vi "Lab Panel V5.26.vi"() -> ()   [LabVIEW 2017] (continued)
                        n2902 = local write "MAIL SETTINGS"(w5260) -> ()
                      }
                    }
                  }
                }
              }
              frame #1 {
                # "mail report"
                n2903 = stacked-sequence {
                  seq-local: [_ w5320 _ _] -> [_ _ _ w5510]
                  seq-local: [_ _ w5423 _] -> [_ _ _ w5500]
                  seq-local: [w5287 _ _ _] -> [_ w5337 _ _]
                  seq-local: [w5286 _ _ _] -> [_ w5336 _ _]
                  seq-local: [w5284 _ _ _] -> [_ w5334 _ _]
                  seq-local: [w5285 _ _ _] -> [_ w5335 _ _]
                  seq-local: [w5283 _ _ _] -> [_ w5333 _ _]
                  seq-local: [w5282 _ _ _] -> [_ w5328 _ _]
                  seq-local: [w5281 _ _ _] -> [_ w5329 _ _]
                  seq-local: [w5280 _ _ _] -> [_ w5330 _ _]
                  seq-local: [w5279 _ _ _] -> [_ w5331 _ _]
                  seq-local: [w5278 _ _ _] -> [_ w5332 _ _]
                  tunnel: w5277 -> [_ _ _ w5511]
                  tunnel: w5276 -> [_ _ _ w5494]
                  tunnel: w5275 -> [_ _ _ w5508]
                  tunnel: w5274 -> [_ _ _ w5507]
                  tunnel: w5273 -> [w5318 _ _ w5502]
                  tunnel: w5272 -> [_ _ w5453 _]
                  tunnel: w5271 -> [_ _ w5450 _]
                  tunnel: w5270 -> [_ _ w5449 _]
                  tunnel: w5269 -> [_ _ w5448 _]
                  tunnel: w5268 -> [_ _ w5447 _]
                  tunnel: w5267 -> [_ _ w5446 _]
                  tunnel: w5266 -> [_ _ w5445 _]
                  tunnel: w5265 -> [_ _ w5444 _]
                  tunnel: w5264 -> [_ _ w5443 _]
                  tunnel: w5263 -> [_ _ w5442 _]
                  frame #0 {
                    n2904 = case shown="False" w5318 {
                      frame False {
                        n2905 = local write "mail control"("") -> ()
                      }
                      frame True {
                      }
                    }
                    n2906 = local read "SET LAB01-1"() -> (w5317:T5)
                    n2907 = local read "SET LAB01-2"() -> (w5316:T5)
                    n2908 = local read "SET LAB02-1"() -> (w5315:T5)
                    n2909 = local read "SET LAB02-2"() -> (w5314:T5)
                    n2910 = local read "SET LAB03-1"() -> (w5313:T5)
                    n2911 = local read "SET LAB04-1"() -> (w5311:T5)
                    n2912 = local read "SET LAB05-1"() -> (w5309:T5)
                    n2913 = local read "SET LAB03-2"() -> (w5312:T5)
                    n2914 = local read "SET LAB04-2"() -> (w5310:T5)
                    n2915 = local read "SET LAB05-2"() -> (w5308:T5)
                    n2916 = Unbundle(w5313) -> ("DESCRIPTION"=w5293:string)  [unwired: 4 out]
                    n2917 = Unbundle(w5312) -> ("DESCRIPTION"=w5292:string)  [unwired: 4 out]
                    n2918 = Unbundle(w5311) -> ("DESCRIPTION"=w5291:string)  [unwired: 4 out]
                    n2919 = Unbundle(w5308) -> ("DESCRIPTION"=w5288:string)  [unwired: 4 out]
                    n2920 = Unbundle(w5314) -> ("DESCRIPTION"=w5294:string)  [unwired: 4 out]
                    n2921 = Unbundle(w5310) -> ("DESCRIPTION"=w5290:string)  [unwired: 4 out]
                    n2922 = Unbundle(w5317) -> ("DESCRIPTION"=w5306:string)  [unwired: 4 out]
                    n2923 = Unbundle(w5315) -> ("DESCRIPTION"=w5295:string)  [unwired: 4 out]
                    n2924 = Unbundle(w5309) -> ("DESCRIPTION"=w5289:string)  [unwired: 4 out]
                    n2925 = Unbundle(w5316) -> ("DESCRIPTION"=w5296:string)  [unwired: 4 out]
                    n2926 = Concatenate Strings("[LAB05-2/", w5288) -> (w5278:string)
                    n2927 = Concatenate Strings("[LAB05-1/", w5289) -> (w5279:string)
                    n2928 = Concatenate Strings("[LAB04-2/", w5290) -> (w5280:string)
                    n2929 = Concatenate Strings("[LAB03-2/", w5292) -> (w5282:string)
                    n2930 = Concatenate Strings("[LAB04-1/", w5291) -> (w5281:string)
                    n2931 = Concatenate Strings("[LAB03-1/", w5293) -> (w5283:string)
                    n2932 = Concatenate Strings("[LAB01-2/", w5296) -> (w5286:string)
                    n2933 = Concatenate Strings("[LAB02-2/", w5294) -> (w5284:string)
                    n2934 = Concatenate Strings("[LAB01-1/", w5306) -> (w5287:string)
                    n2935 = Concatenate Strings("[LAB02-1/", w5295) -> (w5285:string)
                  }
                  frame #1 {
                    w5341 = "/"
                    w5342 = 2.0
                    n2936 = local read "DISP LAB01-2"() -> (w5421:T4)
                    n2937 = local read "DISP LAB01-1"() -> (w5422:T4)
                    n2938 = local read "DISP LAB02-1"() -> (w5420:T4)
                    n2939 = local read "DISP LAB03-2"() -> (w5417:T4)
                    n2940 = local read "DISP LAB02-2"() -> (w5419:T4)
                    n2941 = local read "DISP LAB03-1"() -> (w5418:T4)
                    n2942 = local read "DISP LAB04-2"() -> (w5415:T4)
                    n2943 = local read "DISP LAB04-1"() -> (w5416:T4)
                    n2944 = local read "DISP LAB05-1"() -> (w5414:T4)
                    n2945 = local read "DISP LAB05-2"() -> (w5413:T4)
                    n2946 = Unbundle(w5421) -> ("CYCLE"=w5405:dbl, "MINS"=w5404:dbl, "STATUS"=w5401:string)
                    n2947 = Unbundle(w5422) -> ("CYCLE"=w5410:dbl, "MINS"=w5409:dbl, "STATUS"=w5406:string)
                    n2948 = Unbundle(w5420) -> ("CYCLE"=w5398:dbl, "MINS"=w5397:dbl, "STATUS"=w5396:string)
                    n2949 = Unbundle(w5417) -> ("CYCLE"=w5385:dbl, "MINS"=w5384:dbl, "STATUS"=w5381:string)
                    n2950 = Unbundle(w5418) -> ("CYCLE"=w5390:dbl, "MINS"=w5389:dbl, "STATUS"=w5386:string)
                    n2951 = Unbundle(w5419) -> ("CYCLE"=w5395:dbl, "MINS"=w5394:dbl, "STATUS"=w5391:string)
                    n2952 = Unbundle(w5416) -> ("CYCLE"=w5380:dbl, "MINS"=w5379:dbl, "STATUS"=w5376:string)
                    n2953 = Unbundle(w5415) -> ("CYCLE"=w5375:dbl, "MINS"=w5374:dbl, "STATUS"=w5371:string)
                    n2954 = Unbundle(w5414) -> ("CYCLE"=w5370:dbl, "MINS"=w5369:dbl, "STATUS"=w5366:string)
                    n2955 = Unbundle(w5413) -> ("CYCLE"=w5412:dbl, "MINS"=w5411:dbl, "STATUS"=w5363:string)
                    n2956 = Number To Decimal String(number=w5398) -> (decimal integer string=w5400:string)  [unwired: 1 in]
                    n2957 = Number To Decimal String(number=w5395) -> (decimal integer string=w5393:string)  [unwired: 1 in]
                    n2958 = Number To Decimal String(number=w5390) -> (decimal integer string=w5388:string)  [unwired: 1 in]
                    n2959 = Number To Decimal String(number=w5405) -> (decimal integer string=w5403:string)  [unwired: 1 in]
                    n2960 = Number To Decimal String(number=w5385) -> (decimal integer string=w5383:string)  [unwired: 1 in]
                    n2961 = Number To Decimal String(number=w5410) -> (decimal integer string=w5408:string)  [unwired: 1 in]
                    n2962 = Number To Decimal String(number=w5412) -> (decimal integer string=w5365:string)  [unwired: 1 in]
                    n2963 = Number To Decimal String(number=w5380) -> (decimal integer string=w5378:string)  [unwired: 1 in]
                    n2964 = Number To Decimal String(number=w5375) -> (decimal integer string=w5373:string)  [unwired: 1 in]
                    n2965 = Number To Decimal String(number=w5370) -> (decimal integer string=w5368:string)  [unwired: 1 in]
                    n2966 = Number To Fractional String(number=w5397, precision (6)=w5342) -> (F-format string=w5399:string)  [unwired: 2 in]
                    n2967 = Number To Fractional String(number=w5384, precision (6)=w5342) -> (F-format string=w5382:string)  [unwired: 2 in]
                    n2968 = Number To Fractional String(number=w5394, precision (6)=w5342) -> (F-format string=w5392:string)  [unwired: 2 in]
                    n2969 = Number To Fractional String(number=w5389, precision (6)=w5342) -> (F-format string=w5387:string)  [unwired: 2 in]
                    n2970 = Number To Fractional String(number=w5374, precision (6)=w5342) -> (F-format string=w5372:string)  [unwired: 2 in]
                    n2971 = Number To Fractional String(number=w5379, precision (6)=w5342) -> (F-format string=w5377:string)  [unwired: 2 in]
                    n2972 = Number To Fractional String(number=w5404, precision (6)=w5342) -> (F-format string=w5402:string)  [unwired: 2 in]
                    n2973 = Number To Fractional String(number=w5369, precision (6)=w5342) -> (F-format string=w5367:string)  [unwired: 2 in]
                    n2974 = Number To Fractional String(number=w5409, precision (6)=w5342) -> (F-format string=w5407:string)  [unwired: 2 in]
                    n2975 = Number To Fractional String(number=w5411, precision (6)=w5342) -> (F-format string=w5364:string)  [unwired: 2 in]
                    n2976 = Concatenate Strings(w5341, w5383, w5341, w5382, w5341, w5381) -> (w5357:string)
                    n2977 = Concatenate Strings(w5341, w5378, w5341, w5377, w5341, w5376) -> (w5356:string)
                    n2978 = Concatenate Strings(w5341, w5373, w5341, w5372, w5341, w5371) -> (w5355:string)
                    n2979 = Concatenate Strings(w5341, w5368, w5341, w5367, w5341, w5366) -> (w5354:string)
                    n2980 = Concatenate Strings(w5341, w5365, w5341, w5364, w5341, w5363) -> (w5353:string)
                    n2981 = Concatenate Strings(w5341, w5408, w5341, w5407, w5341, w5406) -> (w5362:string)
                    n2982 = Concatenate Strings(w5341, w5388, w5341, w5387, w5341, w5386) -> (w5358:string)
                    n2983 = Concatenate Strings(w5341, w5403, w5341, w5402, w5341, w5401) -> (w5361:string)
                    n2984 = Concatenate Strings(w5341, w5400, w5341, w5399, w5341, w5396) -> (w5360:string)
                    n2985 = Concatenate Strings(w5341, w5393, w5341, w5392, w5341, w5391) -> (w5359:string)
                    n2986 = Concatenate Strings("]", "\r") -> (w5338:string)
                    n2987 = Concatenate Strings(w5333, w5358, w5338) -> (w5348:string)
                    n2988 = Concatenate Strings(w5335, w5360, w5338) -> (w5350:string)
                    n2989 = Concatenate Strings(w5334, w5359, w5338) -> (w5349:string)
                    n2990 = Concatenate Strings(w5330, w5355, w5338) -> (w5345:string)
                    n2991 = Concatenate Strings(w5331, w5354, w5338) -> (w5346:string)
                    n2992 = Concatenate Strings(w5329, w5356, w5338) -> (w5344:string)
                    n2993 = Concatenate Strings(w5328, w5357, w5338) -> (w5343:string)
                    n2994 = Concatenate Strings(w5332, w5353, w5338) -> (w5347:string)
                    n2995 = Concatenate Strings(w5336, w5361, w5338) -> (w5351:string)
                    n2996 = Concatenate Strings(w5337, w5362, w5338) -> (w5352:string)
                    n2997 = Concatenate Strings(w5352, w5351, w5350, w5349, w5348, w5343, w5344, w5345, w5346, w5347) -> (w5321:string)
                    n2998 = Concatenate Strings("[PANEL/", "DESC/", "CYCLES/", "MINS/", "STATUS]", "\r", w5321) -> (w5320:string)
                    "MAIL REPORT" <- w5320
                    n2999 = global write "Global display 3.vi" "log all"(w5320) -> ()
                  }
                  frame #2 {
                    w5451 = "END"
                    n3000 = local read "mail control"() -> (w5452:string)
                    n3001 = case shown="False" w5447 {
                      tunnel: w5452 -> [w5476 _]
                      tunnel: w5451 -> [w5475 _]
                      tunnel: [w5474 FALSE] -> w5437
                      frame False {
                        n3002 = Equal?(x=w5476, y=w5475) -> (x = y?=w5474:bool)
                      }
                      frame True {
                      }
                    }
                    n3003 = case shown="False" w5453 {
                      tunnel: w5452 -> [w5492 _]
                      tunnel: w5451 -> [w5491 _]
                      tunnel: [w5490 FALSE] -> w5441
                      frame False {
                        n3004 = Equal?(x=w5492, y=w5491) -> (x = y?=w5490:bool)
                      }
                      frame True {
                      }
                    }
                    n3005 = case shown="False" w5450 {
                      tunnel: w5452 -> [w5488 _]
                      tunnel: w5451 -> [w5487 _]
                      tunnel: [w5486 FALSE] -> w5440
                      frame False {
                        n3006 = Equal?(x=w5488, y=w5487) -> (x = y?=w5486:bool)
                      }
                      frame True {
                      }
                    }
                    n3007 = case shown="False" w5448 {
                      tunnel: w5452 -> [w5480 _]
                      tunnel: w5451 -> [w5479 _]
                      tunnel: [w5478 FALSE] -> w5438
                      frame False {
                        n3008 = Equal?(x=w5480, y=w5479) -> (x = y?=w5478:bool)
                      }
                      frame True {
                      }
                    }
                    n3009 = case shown="False" w5449 {
                      tunnel: w5452 -> [w5484 _]
                      tunnel: w5451 -> [w5483 _]
                      tunnel: [w5482 FALSE] -> w5439
                      frame False {
                        n3010 = Equal?(x=w5484, y=w5483) -> (x = y?=w5482:bool)
                      }
                      frame True {
                      }
                    }
                    n3011 = Or(x=w5439, y=w5438) -> (x .or. y?=w5430:bool)
                    n3012 = Or(x=w5441, y=w5440) -> (x .or. y?=w5431:bool)
                    n3013 = Or(x=w5431, y=w5430) -> (x .or. y?=w5426:bool)
                    n3014 = case shown="False" w5443 {
                      tunnel: w5452 -> [w5460 _]
                      tunnel: w5451 -> [w5459 _]
                      tunnel: [w5458 FALSE] -> w5432
                      frame False {
                        n3015 = Equal?(x=w5460, y=w5459) -> (x = y?=w5458:bool)
                      }
                      frame True {
                      }
                    }
                    n3016 = case shown="False" w5442 {
                      tunnel: w5452 -> [w5456 _]
                      tunnel: w5451 -> [w5455 _]
                      tunnel: [w5454 FALSE] -> w5436
                      frame False {
                        n3017 = Equal?(x=w5456, y=w5455) -> (x = y?=w5454:bool)
                      }
                      frame True {
                      }
                    }
                    n3018 = case shown="False" w5444 {
                      tunnel: w5452 -> [w5464 _]
                      tunnel: w5451 -> [w5463 _]
                      tunnel: [w5462 FALSE] -> w5433
                      frame False {
                        n3019 = Equal?(x=w5464, y=w5463) -> (x = y?=w5462:bool)
                      }
                      frame True {
                      }
                    }
                    n3020 = case shown="False" w5446 {
                      tunnel: w5452 -> [w5472 _]
                      tunnel: w5451 -> [w5471 _]
                      tunnel: [w5470 FALSE] -> w5435
                      frame False {
                        n3021 = Equal?(x=w5472, y=w5471) -> (x = y?=w5470:bool)
                      }
                      frame True {
                      }
                    }
                    n3022 = case shown="False" w5445 {
                      tunnel: w5452 -> [w5468 _]
                      tunnel: w5451 -> [w5467 _]
                      tunnel: [w5466 FALSE] -> w5434
                      frame False {
                        n3023 = Equal?(x=w5468, y=w5467) -> (x = y?=w5466:bool)
                      }
                      frame True {
                      }
                    }
                    n3024 = Or(x=w5435, y=w5434) -> (x .or. y?=w5429:bool)
                    n3025 = Or(x=w5433, y=w5432) -> (x .or. y?=w5428:bool)
                    n3026 = Or(x=w5436, y=w5437) -> (x .or. y?=w5424:bool)
                    n3027 = Or(x=w5429, y=w5428) -> (x .or. y?=w5427:bool)
                    n3028 = Or(x=w5426, y=w5427) -> (x .or. y?=w5425:bool)
                    n3029 = Or(x=w5425, y=w5424) -> (x .or. y?=w5423:bool)
                  }
                  frame #3 {
                    n3030 = local read "on loops"() -> (w5506:dbl)
                    n3031 = local read "jig cycle"() -> (w5503:dbl)
                    n3032 = local read "Send Mail Now"() -> (w5497:bool)
                    n3033 = Add(x=w5506, y=5.0) -> (x+y=w5504:dbl)
                    n3034 = Equal?(x=w5503, y=w5504) -> (x = y?=w5498:bool)
                    n3035 = And(x=w5498, y=w5497) -> (x .and. y?=w5496:bool)
                    n3036 = And(x=w5502, y=w5498) -> (x .and. y?=w5501:bool)
                    n3037 = And(x=w5501, y=w5500) -> (x .and. y?=w5499:bool)
                    n3038 = Or(x=w5499, y=w5496) -> (x .or. y?=w5495:bool)
                    n3039 = case shown="True" w5495 {
                      tunnel: w5511 -> [_ w5517]
                      tunnel: w5510 -> [_ w5516]
                      tunnel: "Lab Panel Test Status" -> [_ w5515]
                      tunnel: w5508 -> [_ w5514]
                      tunnel: w5507 -> [_ w5513]
                      tunnel: w5494 -> [_ w5512]
                      frame False {
                      }
                      frame True {
                        n3040 = stacked-sequence {
                          tunnel: w5517 -> [w5525 _]
                          tunnel: w5516 -> [w5524 _]
                          tunnel: w5515 -> [w5523 _]
                          tunnel: w5514 -> [w5522 _]
                          tunnel: w5513 -> [w5521 _]
                          tunnel: w5512 -> [w5520 _]
                          frame #0 {
                            n3041 = call "Lab Send Mail Test.vi"("TO:"=w5525, "subject"=w5523, "from"=w5521, "out going server"=w5522, "message"=w5524) -> ("error out"=w5519:errorcluster)  [unwired: 10 in]
                            n3042 = Bundle(cluster=w5520, "mail error"=w5519) -> (w5518:T7)  [unwired: 6 in]
                            n3043 = local write "MAIL SETTINGS"(w5518) -> ()
                          }
                          frame #1 {
                            n3044 = local write "mail control"("") -> ()
                            n3045 = local write "Send Mail Now"(FALSE) -> ()
                          }
                        }
                      }
                    }
                  }
                }
              }
            }
          }
          frame #20 {
            # "save jig cycle values once all run switches are off"
            n3046 = stacked-sequence {
              tunnel: w5537 -> [_ w5566]
              tunnel: w5536 -> [_ w5565]
              tunnel: w5535 -> [_ w5564]
              tunnel: w5534 -> [_ w5563]
              tunnel: w5533 -> [_ w5562]
              tunnel: w5532 -> [_ w5561]
              tunnel: w5531 -> [_ w5560]
              tunnel: w5530 -> [_ w5559]
              tunnel: w5529 -> [_ w5558]
              tunnel: w5528 -> [_ w5557]
              frame #0 {
              }
              frame #1 {
                n3047 = Not(x=w5557) -> (.not. x?=w5540:bool)
                n3048 = Not(x=w5565) -> (.not. x?=w5555:bool)
                n3049 = Not(x=w5562) -> (.not. x?=w5550:bool)
                n3050 = Not(x=w5560) -> (.not. x?=w5546:bool)
                n3051 = Not(x=w5558) -> (.not. x?=w5542:bool)
                n3052 = Not(x=w5566) -> (.not. x?=w5556:bool)
                n3053 = Not(x=w5564) -> (.not. x?=w5554:bool)
                n3054 = Not(x=w5561) -> (.not. x?=w5548:bool)
                n3055 = Not(x=w5563) -> (.not. x?=w5552:bool)
                n3056 = Not(x=w5559) -> (.not. x?=w5544:bool)
                n3057 = local read "Save JC"() -> (w5568:bool)
                n3058 = And(x=w5556, y=w5555) -> (x .and. y?=w5553:bool)
                n3059 = And(x=w5553, y=w5554) -> (x .and. y?=w5551:bool)
                n3060 = And(x=w5551, y=w5552) -> (x .and. y?=w5549:bool)
                n3061 = And(x=w5549, y=w5550) -> (x .and. y?=w5547:bool)
                n3062 = And(x=w5547, y=w5548) -> (x .and. y?=w5545:bool)
                n3063 = And(x=w5545, y=w5546) -> (x .and. y?=w5543:bool)
                n3064 = And(x=w5543, y=w5544) -> (x .and. y?=w5541:bool)
                n3065 = And(x=w5541, y=w5542) -> (x .and. y?=w5539:bool)
                n3066 = And(x=w5539, y=w5540) -> (x .and. y?=w5538:bool)
                n3067 = And(x=w5538, y=w5568) -> (x .and. y?=w5567:bool)
                n3068 = case shown="True" w5567 {
                  tunnel: w5538 -> [w5569 _]
                  frame False {
                    n3069 = case shown="False" w5569 {
                      frame False {
                        n3070 = local write "Save JC"(TRUE) -> ()
                      }
                      frame True {
                      }
                    }
                  }
                  frame True {
                    n3071 = stacked-sequence {
                      frame #0 {
                        n3072 = String To Path(string="c:\\crabtree\\Jig Cycles\\") -> (path=w5581:path)
                        n3073 = Build Path(base path=w5581, name or relative path="jigcycles.bin") -> (appended path=w5579:path)
                        n3074 = Create Folder(path (use dialog)=w5581) -> (error out=w5583:errorcluster)  [unwired: 2 in, 2 out]
                        n3075 = local read "JIG RELAY CYCLES"() -> (w5573:T8)
                        n3076 = call <vilib>:"Clear Errors.vi"("error in (no error)"=w5583) -> ()  [unwired: 5 in, 2 out]
                        n3077 = local write "Save JC"(FALSE) -> ()
                        n3078 = Open/Create/Replace File(file path (use dialog)=w5579, operation (0:open)=T17."replace or create") -> (refnum out=w5577:refnum<file>, error out=w5578:errorcluster)  [unwired: 4 in, 1 out]
                        n3079 = Write to Binary File(file (use dialog)=w5577, data=w5573, error in=w5578) -> (refnum out=w5576:refnum<file>, error out=w5575:errorcluster)  [unwired: 3 in, 1 out]
                        n3080 = Close File(refnum=w5576, error in=w5575) -> (error out=w5574:errorcluster)  [unwired: 1 out]
                        n3081 = local write "data file error"(w5574) -> ()
                      }
                      frame #1 {
                        n3082 = local read "JIG RELAY CYCLES"() -> (w5606:T8)
                        n3083 = Unbundle By Name(w5606) -> ("LAB01-1"=w5601:dbl, "LAB01-2"=w5600:dbl, "LAB02-1"=w5598:dbl, "LAB02-2"=w5597:dbl, "LAB03-1"=w5595:dbl, "LAB03-2"=w5592:dbl, "LAB04-1"=w5591:dbl, "LAB04-2"=w5589:dbl, "LAB05-1"=w5587:dbl, "LAB05-2"=w5585:dbl)
                        n3084 = stacked-sequence {
                          tunnel: w5601 -> [w5609 _ _ _ _ _ _ _ _ _]
                          tunnel: 1000000 -> [w5612 w5622 w5632 w5642 w5652 w5662 w5672 w5682 w5692 w5702]
                          tunnel: [w5610 _ _ _ _ _ _ _ _ _] -> w5604
                          tunnel: "TEST STATION HAS REACHED 1 MILLION CYCLES, REPLACE  CONTROL RELAYS" -> [w5608 w5620 w5630 w5640 w5650 w5660 w5670 w5680 w5690 w5700]
                          tunnel: [_ w5619 _ _ _ _ _ _ _ _] -> w5602
                          tunnel: w5600 -> [_ w5618 _ _ _ _ _ _ _ _]
                          tunnel: [_ _ w5629 _ _ _ _ _ _ _] -> w5599
                          tunnel: w5598 -> [_ _ w5628 _ _ _ _ _ _ _]
                          tunnel: w5597 -> [_ _ _ w5639 _ _ _ _ _ _]
                          tunnel: [_ _ _ w5638 _ _ _ _ _ _] -> w5596
                          tunnel: w5595 -> [_ _ _ _ w5649 _ _ _ _ _]
                          tunnel: [_ _ _ _ w5648 _ _ _ _ _] -> w5594
                          tunnel: [_ _ _ _ _ w5659 _ _ _ _] -> w5593
                          tunnel: w5592 -> [_ _ _ _ _ w5658 _ _ _ _]
                          tunnel: w5591 -> [_ _ _ _ _ _ w5669 _ _ _]
                          tunnel: [_ _ _ _ _ _ w5668 _ _ _] -> w5590
                          tunnel: w5589 -> [_ _ _ _ _ _ _ w5679 _ _]
                          tunnel: [_ _ _ _ _ _ _ w5678 _ _] -> w5588
                          tunnel: w5587 -> [_ _ _ _ _ _ _ _ w5689 _]
                          tunnel: [_ _ _ _ _ _ _ _ w5688 _] -> w5586
                          tunnel: w5585 -> [_ _ _ _ _ _ _ _ _ w5699]
                          tunnel: [_ _ _ _ _ _ _ _ _ w5698] -> w5584
                          frame #0 {
                            n3085 = Greater?(x=w5609, y=w5612) -> (0:w5611:bool)
                            n3086 = case shown="True" w5611 {
                              tunnel: [w5613 0] -> w5610
                              tunnel: w5609 -> [w5613 _]
                              tunnel: w5608 -> [_ w5614]
                              frame False {
                              }
                              frame True {
                                n3087 = Concatenate Strings("LA01-1 ", w5614) -> (w5617:string)
                                n3088 = One Button Dialog(message=w5617) -> ()  [unwired: 1 in, 1 out]
                              }
                            }
                          }
                          frame #1 {
                            n3089 = Greater?(x=w5618, y=w5622) -> (0:w5621:bool)
                            n3090 = case shown="True" w5621 {
                              tunnel: [w5623 0] -> w5619
                              tunnel: w5618 -> [w5623 _]
                              tunnel: w5620 -> [_ w5624]
                              frame False {
                              }
                              frame True {
                                n3091 = Concatenate Strings("LA01-2 ", w5624) -> (w5627:string)
                                n3092 = One Button Dialog(message=w5627) -> ()  [unwired: 1 in, 1 out]
                              }
                            }
                          }
                          frame #2 {
                            n3093 = Greater?(x=w5628, y=w5632) -> (0:w5631:bool)
                            n3094 = case shown="True" w5631 {
                              tunnel: [w5633 0] -> w5629
                              tunnel: w5628 -> [w5633 _]
                              tunnel: w5630 -> [_ w5634]
                              frame False {
                              }
                              frame True {
                                n3095 = Concatenate Strings("LA02-1 ", w5634) -> (w5637:string)
                                n3096 = One Button Dialog(message=w5637) -> ()  [unwired: 1 in, 1 out]
                              }
                            }
                          }
                          frame #3 {
                            n3097 = Greater?(x=w5639, y=w5642) -> (0:w5641:bool)
                            n3098 = case shown="True" w5641 {
                              tunnel: [w5643 0] -> w5638
                              tunnel: w5639 -> [w5643 _]
                              tunnel: w5640 -> [_ w5644]
                              frame False {
                              }
                              frame True {
                                n3099 = Concatenate Strings("LA02-2 ", w5644) -> (w5647:string)
                                n3100 = One Button Dialog(message=w5647) -> ()  [unwired: 1 in, 1 out]
                              }
                            }
                          }
                          frame #4 {
                            n3101 = Greater?(x=w5649, y=w5652) -> (0:w5651:bool)
                            n3102 = case shown="True" w5651 {
                              tunnel: [w5653 0] -> w5648
                              tunnel: w5649 -> [w5653 _]
                              tunnel: w5650 -> [_ w5654]
                              frame False {
                              }
                              frame True {
                                n3103 = Concatenate Strings("LA03-1 ", w5654) -> (w5657:string)
                                n3104 = One Button Dialog(message=w5657) -> ()  [unwired: 1 in, 1 out]
                              }
                            }
                          }
                          frame #5 {
                            n3105 = Greater?(x=w5658, y=w5662) -> (0:w5661:bool)
                            n3106 = case shown="True" w5661 {
                              tunnel: [w5663 0] -> w5659
                              tunnel: w5658 -> [w5663 _]
                              tunnel: w5660 -> [_ w5664]
                              frame False {
                              }
                              frame True {
                                n3107 = Concatenate Strings("LA03-2 ", w5664) -> (w5667:string)
                                n3108 = One Button Dialog(message=w5667) -> ()  [unwired: 1 in, 1 out]
                              }
                            }
                          }
                          frame #6 {
                            n3109 = Greater?(x=w5669, y=w5672) -> (0:w5671:bool)
                            n3110 = case shown="True" w5671 {
                              tunnel: [w5673 0] -> w5668
                              tunnel: w5669 -> [w5673 _]
                              tunnel: w5670 -> [_ w5674]
                              frame False {
                              }
                              frame True {
                                n3111 = Concatenate Strings("LA04-1 ", w5674) -> (w5677:string)
                                n3112 = One Button Dialog(message=w5677) -> ()  [unwired: 1 in, 1 out]
                              }
                            }
                          }
                          frame #7 {
                            n3113 = Greater?(x=w5679, y=w5682) -> (0:w5681:bool)
                            n3114 = case shown="True" w5681 {
                              tunnel: [w5683 0] -> w5678
                              tunnel: w5679 -> [w5683 _]
                              tunnel: w5680 -> [_ w5684]
                              frame False {
                              }
                              frame True {
                                n3115 = Concatenate Strings("LA04-2 ", w5684) -> (w5687:string)
                                n3116 = One Button Dialog(message=w5687) -> ()  [unwired: 1 in, 1 out]
                              }
                            }
                          }
                          frame #8 {
                            n3117 = Greater?(x=w5689, y=w5692) -> (0:w5691:bool)
                            n3118 = case shown="True" w5691 {
                              tunnel: [w5693 0] -> w5688
                              tunnel: w5689 -> [w5693 _]
                              tunnel: w5690 -> [_ w5694]
                              frame False {
                              }
                              frame True {
                                n3119 = Concatenate Strings("LA05-1 ", w5694) -> (w5697:string)
                                n3120 = One Button Dialog(message=w5697) -> ()  [unwired: 1 in, 1 out]
                              }
                            }
                          }
                          frame #9 {
                            n3121 = Greater?(x=w5699, y=w5702) -> (0:w5701:bool)
                            n3122 = case shown="True" w5701 {
                              tunnel: [w5703 0] -> w5698
                              tunnel: w5699 -> [w5703 _]
                              tunnel: w5700 -> [_ w5704]
                              frame False {
                              }
                              frame True {
                                n3123 = Concatenate Strings("LA05-2 ", w5704) -> (w5707:string)
                                n3124 = One Button Dialog(message=w5707) -> ()  [unwired: 1 in, 1 out]
                              }
                            }
                          }
                        }
                        n3125 = Bundle By Name(cluster=w5606, "LAB01-1"=w5604, "LAB01-2"=w5602, "LAB02-1"=w5599, "LAB02-2"=w5596, "LAB03-1"=w5594, "LAB03-2"=w5593, "LAB04-1"=w5590, "LAB04-2"=w5588, "LAB05-1"=w5586, "LAB05-2"=w5584) -> (w5605:T8)
                        n3126 = local write "JIG RELAY CYCLES"(w5605) -> ()
                      }
                    }
                  }
                }
              }
            }
          }
          frame #21 {
            # "get temperature values"
            n3127 = local read "Simulate"() -> (w5720:bool)
            n3128 = local read "Temp Test Cal"() -> (w5717:dbl)
            n3129 = stacked-sequence {
              seq-local: [w5722 _] -> [_ w5767]
              tunnel: w5720 -> [_ w5780]
              tunnel: T14 {"1  (A) cal"=1.0, "1 (V) cal"=1.0, "1 (PF) cal"=1.0, "1 (TL) cal"=1.0, "1 (TN) cal"=1.0, "2 (A) cal"=1.0, "2 (V) cal"=1.0, "2 (PF) cal"=1.0, "2 (TL) cal"=1.0, "2 (TN) cal"=1.0} ("CAL LAB01") -> [_ w5779]
              tunnel: w5718 -> [_ w5778]
              tunnel: w5717 -> [_ w5777]
              tunnel: w5716 -> [_ w5776]
              tunnel: w5715 -> [_ w5775]
              tunnel: w5714 -> [_ w5774]
              tunnel: w5713 -> [_ w5773]
              tunnel: w5712 -> [_ w5772]
              tunnel: w5711 -> [_ w5771]
              tunnel: w5710 -> [_ w5770]
              tunnel: w5709 -> [_ w5769]
              tunnel: w5708 -> [_ w5768]
              frame #0 {
                # "only get temperature from initial valid temperature circuits"
                n3130 = local read "Select COM port"() -> (w5730:refnum<visa-resource-name>)
                "COM port" <- w5730
                n3131 = global write "Global 1.vi" "COM port"(w5730) -> ()
                n3132 = local read "Temp read loop"() -> (w5727:dbl)
                n3133 = global write "Global 1.vi" "tmp dly lps"("Temp Delay Lps") -> ()
                n3134 = global write "Global 1.vi" "dly value"("Temp Value") -> ()
                n3135 = local read "jig cycle"() -> (w5731:dbl)
                n3136 = local read "on loops"() -> (w5733:dbl)
                n3137 = Equal?(x=w5727, y=1) -> (x = y?=w5724:bool)
                n3138 = Add(x=w5733, y=6) -> (x+y=w5734:dbl)
                n3139 = Equal?(x=w5731, y=w5734) -> (x = y?=w5725:bool)
                n3140 = And(x=w5725, y=w5724) -> (x .and. y?=w5723:bool)
                n3141 = Or(x=w5723, y="Read Temp") -> (x .or. y?=w5722:bool)
                n3142 = case shown="True" w5722 {
                  frame False {
                  }
                  frame True {
                    n3143 = local read "Simulate"() -> (w5736:bool)
                    n3144 = local write "TEMP"(TRUE) -> ()
                    n3145 = local write "Read Temp"(FALSE) -> ()
                    n3146 = stacked-sequence {
                      tunnel: 1.0 -> [_ _ _ _ w5766]
                      tunnel: w5736 -> [_ _ _ _ w5765]
                      frame #0 {
                        # "only switch relay on to reset temp circuits if busy testing"
                        n3147 = disable-structure shown="Disabled" {
                          frame Disabled {
                            n3148 = local read "Any Test Running"() -> ()  [unwired: 1 out]
                          }
                          frame Enabled {
                          }
                        }
                        n3149 = local read "USB OUT 0"() -> (w5740:bool[])
                        n3150 = local read "USB OUT 2"() -> (w5742:bool[])
                        n3151 = local read "USB OUT 1"() -> (w5741:bool[])
                        n3152 = Insert Into Array(array=w5742, index=7, new element=TRUE) -> (w5743:bool[])
                        n3153 = call "sub vi - Drive Relays All v6.vi"("Array #2"=w5743, "Array #1"=w5741, "Array #0"=w5740) -> ()  [unwired: 8 in, 1 out]
                      }
                      frame #1 {
                        # "time delay"
                        n3154 = Wait (ms)(milliseconds to wait=500) -> ()  [unwired: 1 out]
                      }
                      frame #2 {
                        # "switch relay off"
                        n3155 = local read "USB OUT 0"() -> (w5746:bool[])
                        n3156 = local read "USB OUT 2"() -> (w5748:bool[])
                        n3157 = local read "USB OUT 1"() -> (w5747:bool[])
                        n3158 = Insert Into Array(array=w5748, index=7, new element=FALSE) -> (w5749:bool[])
                        n3159 = call "sub vi - Drive Relays All v6.vi"("Array #2"=w5749, "Array #1"=w5747, "Array #0"=w5746) -> ()  [unwired: 8 in, 1 out]
                      }
                      frame #3 {
                        # "time delay"
                        n3160 = Wait (ms)(milliseconds to wait=300) -> ()  [unwired: 1 out]
                      }
                      frame #4 {
                        # "read all valid temp circuits"
                        n3161 = local read "LAB01-TP"() -> (w5758:bool)
                        n3162 = local read "LAB03-TP"() -> (w5756:bool)
                        n3163 = local read "LAB02-TP"() -> (w5757:bool)
                        n3164 = local read "LAB04-TP"() -> (w5755:bool)
                        n3165 = local read "LAB05-TP"() -> (w5759:bool)
                        n3166 = call "sub vi - GET ALL TEMP v7.vi"("LA01-EN"=w5758, "simulate"=w5765, "LA02-EN"=w5757, "LA03-EN"=w5756, "LA04-EN"=w5755, "LA05-EN"=w5759, "Gen Cal Value"=w5766) -> ("LOOP TIME"=→"Read Time":dbl, "LA01 TEMP"=w5764:T25, "LA02 TEMP"=w5763:T25, "LA03 TEMP"=w5762:T25, "LA04 TEMP"=w5761:T25, "error"=→"Error Temp":bool, "LA05 TEMP"=w5760:T25)  [unwired: 1 in, 1 out]
                        n3167 = local write "LAB01 TEMP"(w5764) -> ()
                        n3168 = local write "LAB02 TEMP"(w5763) -> ()
                        n3169 = local write "LAB03 TEMP"(w5762) -> ()
                        n3170 = local write "LAB04 TEMP"(w5761) -> ()
                        n3171 = local write "LAB05 TEMP"(w5760) -> ()
                      }
                    }
                  }
                }
              }
              frame #1 {
                n3172 = case shown="True" w5767 {
                  tunnel: w5780 -> [_ w5793]
                  tunnel: w5779 -> [_ w5792]
                  tunnel: w5778 -> [_ w5791]
                  tunnel: w5777 -> [_ w5790]
                  tunnel: w5776 -> [_ w5789]
                  tunnel: w5775 -> [_ w5788]
                  tunnel: w5774 -> [_ w5787]
                  tunnel: w5773 -> [_ w5786]
                  tunnel: w5772 -> [_ w5785]
                  tunnel: w5771 -> [_ w5784]
                  tunnel: w5770 -> [_ w5783]
                  tunnel: w5769 -> [_ w5782]
                  tunnel: w5768 -> [_ w5781]
                  frame False {
                  }
                  frame True {
                    n3173 = stacked-sequence {
                      tunnel: w5793 -> [_ w5806 w5851 w5896 w5941 w5986]
                      tunnel: w5792 -> [_ w5805 w5850 w5895 w5940 w5985]
                      tunnel: w5791 -> [_ w5795 _ _ _ _]
                      tunnel: w5790 -> [_ w5800 w5849 w5894 w5939 w5984]
                      tunnel: w5789 -> [_ w5794 _ _ _ _]
                      tunnel: w5788 -> [_ _ w5840 _ _ _]
                      tunnel: w5787 -> [_ _ w5839 _ _ _]
                      tunnel: w5786 -> [_ _ _ w5885 _ _]
                      tunnel: w5785 -> [_ _ _ w5884 _ _]
                      tunnel: w5784 -> [_ _ _ _ w5930 _]
                      tunnel: w5783 -> [_ _ _ _ w5929 _]
                      tunnel: w5782 -> [_ _ _ _ _ w5975]
                      tunnel: w5781 -> [_ _ _ _ _ w5974]
                      frame #0 {
                      }
                      frame #1 {
                        n3174 = case shown="False" w5806 {
                          tunnel: [w5837 w5838] -> w5822
                          tunnel: w5805 -> [_ w5838]
                          frame False {
                            n3175 = local read "CAL LAB01"() -> (w5837:T14)
                          }
                          frame True {
                          }
                        }
                        n3176 = local read "TEMP LA01"() -> (w5813:T9)
                        n3177 = local read "LAB01 TEMP"() -> (w5812:T12)
                        n3178 = call "sub vi - temperature delay v3.vi"("2-run"=w5794, "1-run"=w5795, "temp values IN"=w5813, "temp signals"=w5812) -> ("T2-N"=w5808:dbl, "T2-L"=w5809:dbl, "T1-N"=w5810:dbl, "T1-L"=w5811:dbl, "temp values OUT"=w5807:T44)  [unwired: 3 in]
                        n3179 = Unbundle By Name(w5822) -> ("1 (TL) cal"=w5817:dbl, "1 (TN) cal"=w5816:dbl, "2 (TL) cal"=w5815:dbl, "2 (TN) cal"=w5814:dbl)  [unwired: 6 out]
                        n3180 = local write "TEMP LA01"(w5807) -> ()
                        n3181 = Multiply(x=w5811, y=w5817) -> (x*y=w5804:dbl)
                        n3182 = Multiply(x=w5810, y=w5816) -> (x*y=w5802:dbl)
                        n3183 = Multiply(x=w5809, y=w5815) -> (x*y=w5799:dbl)
                        n3184 = Multiply(x=w5808, y=w5814) -> (x*y=w5798:dbl)
                        n3185 = case shown="True" w5795 {
                          tunnel: w5804 -> [w5831 w5836]
                          tunnel: w5800 -> [_ w5834]
                          tunnel: [w5831 w5835] -> w5803
                          tunnel: w5802 -> [w5830 w5833]
                          tunnel: [w5830 w5832] -> w5801
                          frame False {
                          }
                          frame True {
                            n3186 = Multiply(x=w5834, y=w5833) -> (x*y=w5832:dbl)
                            n3187 = Multiply(x=w5834, y=w5836) -> (x*y=w5835:dbl)
                          }
                        }
                        n3188 = case shown="True" w5794 {
                          tunnel: w5799 -> [w5824 w5829]
                          tunnel: w5800 -> [_ w5827]
                          tunnel: [w5824 w5828] -> w5797
                          tunnel: w5798 -> [w5823 w5826]
                          tunnel: [w5823 w5825] -> w5796
                          frame False {
                          }
                          frame True {
                            n3189 = Multiply(x=w5827, y=w5826) -> (x*y=w5825:dbl)
                            n3190 = Multiply(x=w5827, y=w5829) -> (x*y=w5828:dbl)
                          }
                        }
                        n3191 = local read "SIG LAB01-2"() -> (w5819:T2)
                        n3192 = local read "SIG LAB01-1"() -> (w5821:T2)
                        n3193 = Bundle By Name(cluster=w5821, "Tmp Live"=w5803, "Tmp Neut"=w5801) -> (w5820:T2)
                        n3194 = Bundle By Name(cluster=w5819, "Tmp Live"=w5797, "Tmp Neut"=w5796) -> (w5818:T2)
                        n3195 = local write "SIG LAB01-1"(w5820) -> ()
                        n3196 = local write "SIG LAB01-2"(w5818) -> ()
                      }
                      frame #2 {
                        n3197 = case shown="True" w5851 {
                          tunnel: [w5882 w5883] -> w5867
                          tunnel: w5850 -> [_ w5883]
                          frame False {
                            n3198 = local read "CAL LAB02"() -> (w5882:T15)
                          }
                          frame True {
                          }
                        }
                        n3199 = local read "LAB02 TEMP"() -> (w5858:T12)
                        n3200 = local read "TEMP LA02"() -> (w5857:T9)
                        n3201 = call "sub vi - temperature delay v3.vi"("2-run"=w5839, "1-run"=w5840, "temp values IN"=w5857, "temp signals"=w5858) -> ("T2-N"=w5852:dbl, "T2-L"=w5853:dbl, "T1-N"=w5854:dbl, "T1-L"=w5855:dbl, "temp values OUT"=w5856:T44)  [unwired: 3 in]
                        n3202 = Unbundle By Name(w5867) -> ("1 (TL) cal"=w5862:dbl, "1 (TN) cal"=w5861:dbl, "2 (TL) cal"=w5860:dbl, "2 (TN) cal"=w5859:dbl)  [unwired: 6 out]
                        n3203 = local write "TEMP LA02"(w5856) -> ()
                        n3204 = Multiply(x=w5855, y=w5862) -> (x*y=w5848:dbl)
                        n3205 = Multiply(x=w5854, y=w5861) -> (x*y=w5847:dbl)
                        n3206 = Multiply(x=w5853, y=w5860) -> (x*y=w5844:dbl)
                        n3207 = Multiply(x=w5852, y=w5859) -> (x*y=w5843:dbl)
                        n3208 = case shown="True" w5840 {
                          tunnel: w5848 -> [w5876 w5881]
                          tunnel: w5849 -> [_ w5879]
                          tunnel: [w5876 w5880] -> w5846
                          tunnel: w5847 -> [w5875 w5878]
                          tunnel: [w5875 w5877] -> w5845
                          frame False {
                          }
                          frame True {
                            n3209 = Multiply(x=w5879, y=w5878) -> (x*y=w5877:dbl)
                            n3210 = Multiply(x=w5879, y=w5881) -> (x*y=w5880:dbl)
                          }
                        }
                        n3211 = case shown="True" w5839 {
                          tunnel: w5844 -> [w5869 w5874]
                          tunnel: w5849 -> [_ w5872]
                          tunnel: [w5869 w5873] -> w5842
                          tunnel: w5843 -> [w5868 w5871]
                          tunnel: [w5868 w5870] -> w5841
                          frame False {
                          }
                          frame True {
                            n3212 = Multiply(x=w5872, y=w5871) -> (x*y=w5870:dbl)
                            n3213 = Multiply(x=w5872, y=w5874) -> (x*y=w5873:dbl)
                          }
                        }
                        n3214 = local read "SIG LAB02-2"() -> (w5864:T2)
                        n3215 = local read "SIG LAB02-1"() -> (w5866:T2)
                        n3216 = Bundle By Name(cluster=w5866, "Tmp Live"=w5846, "Tmp Neut"=w5845) -> (w5865:T2)
                        n3217 = Bundle By Name(cluster=w5864, "Tmp Live"=w5842, "Tmp Neut"=w5841) -> (w5863:T2)
                        n3218 = local write "SIG LAB02-1"(w5865) -> ()
                        n3219 = local write "SIG LAB02-2"(w5863) -> ()
                      }
                      frame #3 {
                        n3220 = case shown="False" w5896 {
                          tunnel: [w5927 w5928] -> w5912
                          tunnel: w5895 -> [_ w5928]
                          frame False {
                            n3221 = local read "CAL LAB03"() -> (w5927:T14)
                          }
                          frame True {
                          }
                        }
                        n3222 = local read "TEMP LA03"() -> (w5902:T9)
                        n3223 = local read "LAB03 TEMP"() -> (w5903:T12)
                        n3224 = call "sub vi - temperature delay v3.vi"("2-run"=w5884, "1-run"=w5885, "temp values IN"=w5902, "temp signals"=w5903) -> ("T2-N"=w5897:dbl, "T2-L"=w5898:dbl, "T1-N"=w5899:dbl, "T1-L"=w5900:dbl, "temp values OUT"=w5901:T44)  [unwired: 3 in]
                        n3225 = Unbundle By Name(w5912) -> ("1 (TL) cal"=w5907:dbl, "1 (TN) cal"=w5906:dbl, "2 (TL) cal"=w5905:dbl, "2 (TN) cal"=w5904:dbl)  [unwired: 6 out]
                        n3226 = local write "TEMP LA03"(w5901) -> ()
                        n3227 = Multiply(x=w5900, y=w5907) -> (x*y=w5893:dbl)
                        n3228 = Multiply(x=w5899, y=w5906) -> (x*y=w5892:dbl)
                        n3229 = Multiply(x=w5898, y=w5905) -> (x*y=w5889:dbl)
                        n3230 = Multiply(x=w5897, y=w5904) -> (x*y=w5888:dbl)
                        n3231 = case shown="True" w5884 {
                          tunnel: w5889 -> [w5914 w5919]
                          tunnel: w5894 -> [_ w5917]
                          tunnel: [w5914 w5918] -> w5887
                          tunnel: w5888 -> [w5913 w5916]
                          tunnel: [w5913 w5915] -> w5886
                          frame False {
                          }
                          frame True {
                            n3232 = Multiply(x=w5917, y=w5916) -> (x*y=w5915:dbl)
                            n3233 = Multiply(x=w5917, y=w5919) -> (x*y=w5918:dbl)
                          }
                        }
                        n3234 = case shown="True" w5885 {
                          tunnel: w5893 -> [w5921 w5926]
                          tunnel: w5894 -> [_ w5924]
                          tunnel: [w5921 w5925] -> w5891
                          tunnel: w5892 -> [w5920 w5923]
                          tunnel: [w5920 w5922] -> w5890
                          frame False {
                          }
                          frame True {
                            n3235 = Multiply(x=w5924, y=w5923) -> (x*y=w5922:dbl)
                            n3236 = Multiply(x=w5924, y=w5926) -> (x*y=w5925:dbl)
                          }
                        }
                        n3237 = local read "SIG LAB03-2"() -> (w5909:T2)
                        n3238 = local read "SIG LAB03-1"() -> (w5911:T2)
                        n3239 = Bundle By Name(cluster=w5911, "Tmp Live"=w5891, "Tmp Neut"=w5890) -> (w5910:T2)
                        n3240 = Bundle By Name(cluster=w5909, "Tmp Live"=w5887, "Tmp Neut"=w5886) -> (w5908:T2)
                        n3241 = local write "SIG LAB03-1"(w5910) -> ()
                        n3242 = local write "SIG LAB03-2"(w5908) -> ()
                      }
                      frame #4 {
                        n3243 = case shown="False" w5941 {
                          tunnel: [w5972 w5973] -> w5957
                          tunnel: w5940 -> [_ w5973]
                          frame False {
                            n3244 = local read "CAL LAB04"() -> (w5972:T14)
                          }
                          frame True {
                          }
                        }
                        n3245 = local read "LAB04 TEMP"() -> (w5947:T12)
                        n3246 = local read "TEMP LA04"() -> (w5948:T9)
